vi "Encoder Test.vi"() -> ()   [LabVIEW 2021]
panel:
  out "x-y":dbl
  out "Mes Pos (mm)":dbl(graph)
  out "RPM":dbl(graph)
  in  "stop":bool
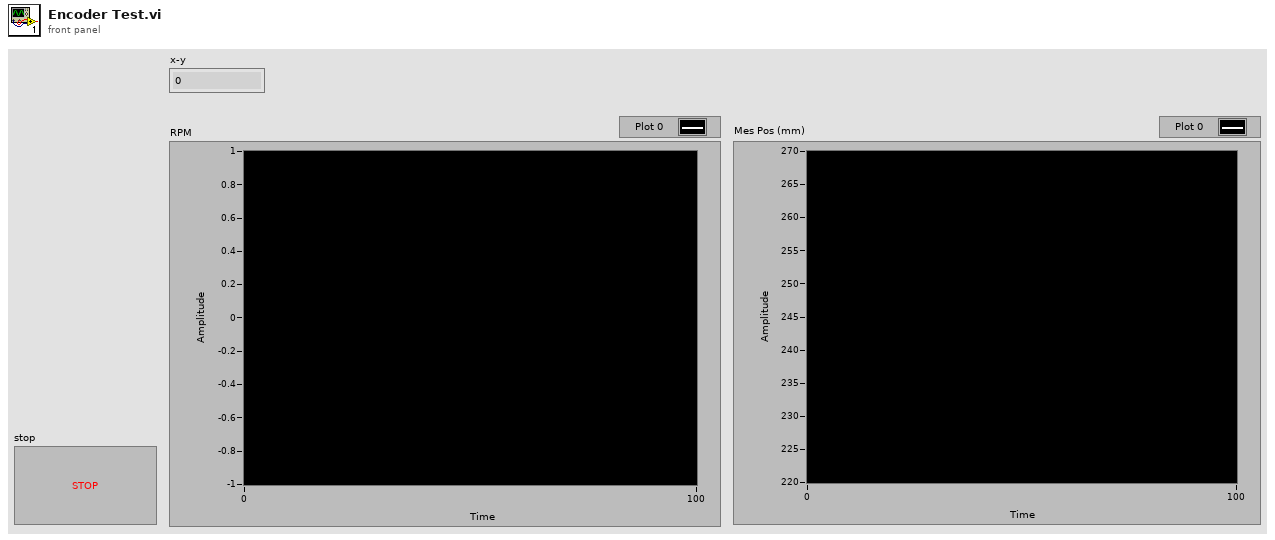
[diagram p1: front panel]
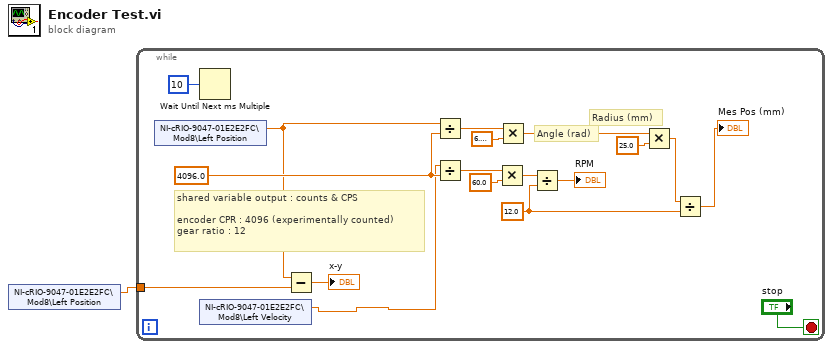
[diagram p0: block diagram]
diagram:
  n1 = shared-variable "NI-cRIO-9047-01E2E2FC\\Mod8\\Left Position"() -> (w1:dbl)  [unwired: 1 in, 1 out]
  n2 = while {
    tunnel: w1 -> [w5]
    stop <- "stop" stop-if-true
    w9 = 12.0 ("y")
    w13 = 4096.0 ("y")
    # "Radius (mm)"
    # "Angle (rad)"
    # "shared variable output : counts & CPS\n\nencoder CPR : 4096 (experimentally counted)\ngear ratio : 12"
    n3 = shared-variable "NI-cRIO-9047-01E2E2FC\\Mod8\\Left Position"() -> (w2:dbl)  [unwired: 1 in, 1 out]
    n4 = Wait Until Next ms Multiple(millisecond multiple=u32 10) -> ()  [unwired: 1 out]
    n5 = shared-variable "NI-cRIO-9047-01E2E2FC\\Mod8\\Left Velocity"() -> (w3:dbl)  [unwired: 1 in, 1 out]
    n6 = Subtract(x=w2, y=w5) -> (x-y=→"x-y":dbl)
    n7 = Divide(x=w2, y=w13) -> (x/y=w15:dbl)
    n8 = Divide(x=w3, y=w13) -> (x/y=w17:dbl)
    n9 = Multiply(x=w17, y=60.0) -> (x*y=w8:dbl)
    n10 = Multiply(x=w15, y=6.283185307179586) -> (x*y=w12:dbl)
    n11 = Divide(x=w8, y=w9) -> (x/y=→"RPM":dbl)
    n12 = Multiply(x=w12, y=25.0) -> (x*y=w10:dbl)
    n13 = Divide(x=w10, y=w9) -> (x/y=→"Mes Pos (mm)":dbl)
  }
